vi "ESP300 CheckErrors.vi"(6 "error in (no error)":errorcluster, 9 "Ressource VISA In":refnum<visa-resource-name>="GPIB0::8::INSTR") -> (0 "error out":errorcluster, 1 "Warning":bool, 2 "Error Message":string, 3 "Ressource VISA Out":refnum<visa-resource-name>="GPIB0::8::INSTR")   [LabVIEW 2019]
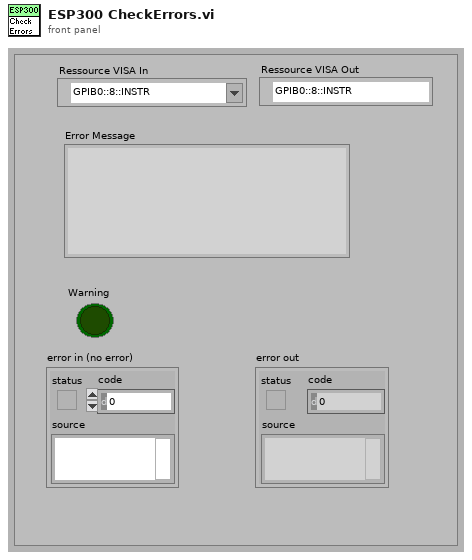
[diagram p1: front panel]
types:
  T1 = enum32{"Invalid", "Standard", "Closed", "Hidden", "Minimized", "Maximized"}
  T2 = enum32{"Bad", "Idle", "Run top level", "Running"}
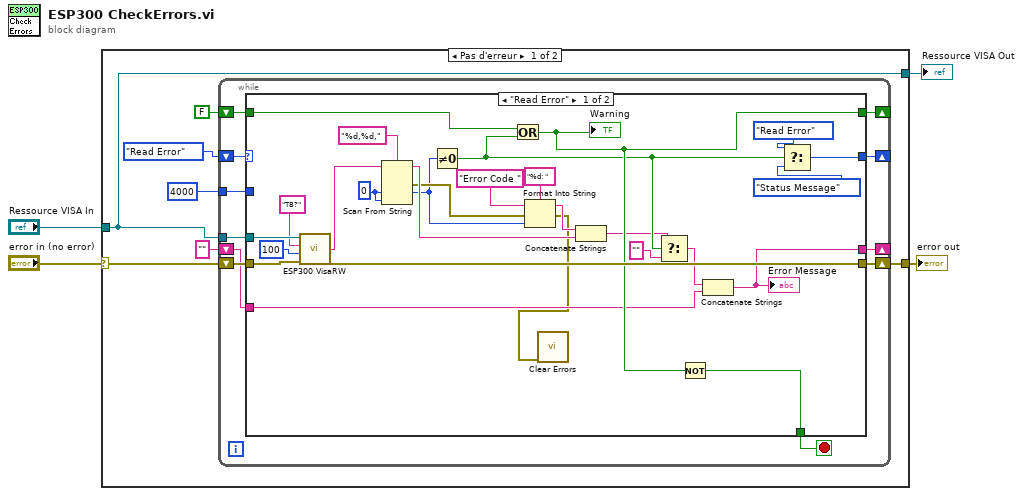
[diagram p0: block diagram]
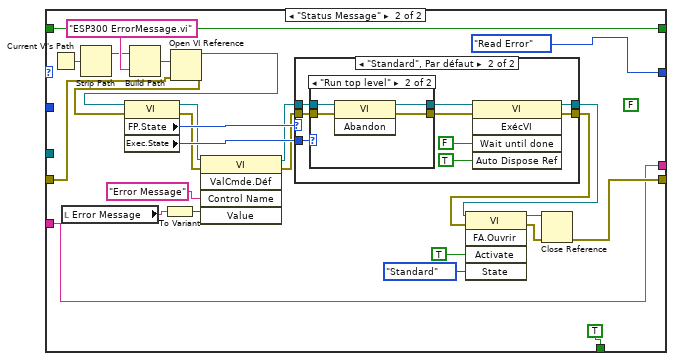
[diagram p2: hidden frame]
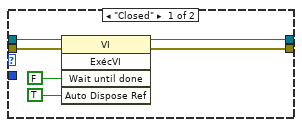
[diagram p3: hidden frame]
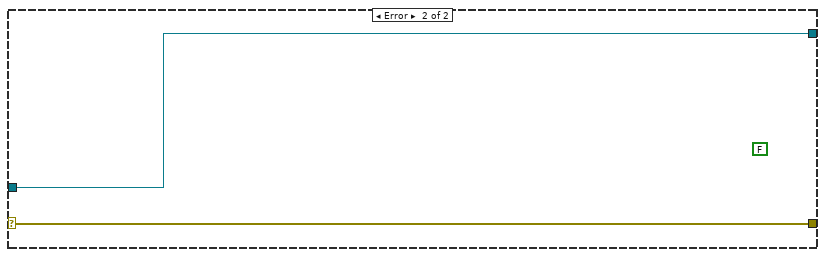
[diagram p5: hidden frame]
diagram:
  n1 = case shown="Pas d'erreur" "error in (no error)" {
    selector: "error in (no error)" -> [w9 w99]
    tunnel: [w10 w99] -> w3
    tunnel: "Ressource VISA In" -> [w7 w98]
    tunnel: [w7 w98] -> w1
    frame No Error {
      n2 = while {
        shift-right: [w17] -> _
        shift-left: enum16{"Read Error", "Status Message"}."Read Error" -> [w22]
        shift-right: [w20] -> w10
        shift-left: w9 -> [w21]
        tunnel: 4000 ("timeout ms (488.2 global)") -> [w19]
        tunnel: w7 -> [w16]
        shift-right: [w15] -> _
        shift-left: FALSE -> [w14]
        shift-right: [w13] -> _
        shift-left: "" -> [w12]
        stop <- w18 stop-if-true
        n3 = case shown="\"Read Error\"" w22 {
          tunnel: w21 -> [w49 w63]
          tunnel: [w48 w64] -> w20
          tunnel: w19 -> [_ _]
          tunnel: [w36 TRUE] -> w18
          tunnel: [w35 enum16{"Read Error", "Status Message"}."Read Error"] -> w17
          tunnel: w16 -> [w47 _]
          tunnel: [w37 w52] -> w15
          tunnel: w14 -> [w38 w52]
          tunnel: [w26 w51] -> w13
          tunnel: w12 -> [w27 w51]
          frame "Read Error" {
            w42 = 0 ("default (0 I32)")
            n4 = call <userlib>:"ESP300 VisaRW.vi"("error in (no error)"=w49, "Nbcaract"=u32 100, "ChaineCom"="TB?", "VISA Rsrc"=w47) -> ("error out"=w48:errorcluster, "ChaineRep"=w43:string)  [unwired: 3 in, 2 out]
            n5 = Scan From String(format string="%d,%d,", input string=w43, default 1=w42, default 2=w42) -> (remaining string=w32:string, error out=w25:errorcluster, output 1=w23:i32)  [unwired: 3 in, 1 out]
            n6 = Not Equal To 0?(x=w23) -> (x != 0?=w31:bool)
            n7 = Or(x=w38, y=w31) -> (x .or. y?=w37:bool)
            "Warning" <- w37
            n8 = Format Into String(format string="%d: ", initial string="Error Code ", error in=w25, w23) -> (resulting string=w39:string, error out=w24:errorcluster)
            n9 = call <vilib>:"Clear Errors.vi"("error in (no error)"=w24) -> ()  [unwired: 5 in, 2 out]
            n10 = Concatenate Strings(w39, w32) -> (w30:string)
            n11 = Select(t=w30, s=w31, f="") -> (s? t:f=w28:string)
            n12 = Not(x=w37) -> (.not. x?=w36:bool)
            n13 = Concatenate Strings(w28, w27) -> (w26:string)
            "Error Message" <- w26
            n14 = Select(t=enum16{"Read Error", "Status Message"}."Read Error", s=w31, f=enum16{"Read Error", "Status Message"}."Status Message") -> (s? t:f=w35:enum16{"Read Error", "Status Message"})
          }
          frame "Status Message" {
            (unwired) FALSE
            n15 = Current VI's Path() -> (path=w74:path)
            n16 = local read "Error Message"() -> (w61:string)
            n17 = Strip Path(path=w74) -> (stripped path=w75:path)  [unwired: 1 out]
            n18 = Build Path(base path=w75, name or relative path="ESP300 ErrorMessage.vi" ("nom ou chemin relatif")) -> (appended path=w70:path)
            n19 = To Variant(anything=w61) -> (Variant=w67:variant)
            n20 = Open VI Reference(vi path=w70, error in (no error)=w63) -> (vi reference=w71:refnum<vi>, error out=w62:errorcluster)  [unwired: 4 in]
            n21 = property class="VI"(reference=w71, error in=w62) -> (reference out=w54:refnum<vi>, error out=w55:errorcluster, "FP.State"=w72:T1, "Exec.State"=w73:T2)
            n22 = invoke class="VI" method="ValCmde.Déf"(reference=w54, error in=w55, "Control Name"="Error Message" ("Nom de la commande"), "Value"=w67) -> (reference out=w56:refnum<vi>, error out=w57:errorcluster)  [unwired: 1 in, 3 out]
            n23 = case shown="\"Standard\", Par défaut" w72 {
              tunnel: [w79 w88] -> w58
              tunnel: w56 -> [w80 w86]
              tunnel: w73 -> [_ w87]
              tunnel: w57 -> [w78 w85]
              tunnel: [w77 w83] -> w59
              frame "Closed" {
                n24 = invoke class="VI" method="ExécVI"(reference=w80, error in=w78, "Wait until done"=FALSE ("Attendre la fin"), "Auto Dispose Ref"=TRUE ("Supprimer la référence automatiquement")) -> (reference out=w79:refnum<vi>, error out=w77:errorcluster)  [unwired: 1 in, 3 out]
              }
              frame "Standard", Default {
                n25 = case shown="\"Run top level\"" w87 {
                  tunnel: [w93 w97] -> w89
                  tunnel: w86 -> [w93 w96]
                  tunnel: w85 -> [w92 w95]
                  tunnel: [w92 w94] -> w84
                  frame "Idle", Default {
                  }
                  frame "Run top level" {
                    n26 = invoke class="VI" method="Abandon"(reference=w96, error in=w95) -> (reference out=w97:refnum<vi>, error out=w94:errorcluster)  [unwired: 1 in, 1 out]
                  }
                }
                n27 = invoke class="VI" method="ExécVI"(reference=w89, error in=w84, "Wait until done"=FALSE ("Attendre la fin"), "Auto Dispose Ref"=TRUE ("Supprimer la référence automatiquement")) -> (reference out=w88:refnum<vi>, error out=w83:errorcluster)  [unwired: 1 in, 3 out]
              }
            }
            n28 = invoke class="VI" method="FA.Ouvrir"(reference=w58, error in=w59, "Activate"=TRUE ("Activer ?"), "State"=T1."Standard" ("État")) -> (reference out=w66:refnum<vi>, error out=w65:errorcluster)  [unwired: 1 in, 3 out]
            n29 = Close Reference(reference=w66, error in (no error)=w65) -> (error out=w64:errorcluster)
          }
        }
      }
    }
    frame Error {
      (unwired) FALSE
    }
  }
  "error out" <- w3
  "Ressource VISA Out" <- w1
